vi "AddTestSuite_NoParent_AddedToRoot.vi"() -> (0 "error out":errorcluster)   [LabVIEW 2019, in "ResultTreeTest.lvlib"]
uses:
  ResultTreeTest.lvlib
  2a6c7ef5-d8ea-4de4-ba7d-c6663dbf2225.vi
  Constraint/IsEqual/Create.vi
  Constraint/IsEqual/IsEqual.lvclass
  ResultTree/ResultTree.lvclass
panel:
  in  "Tree":string(tree)
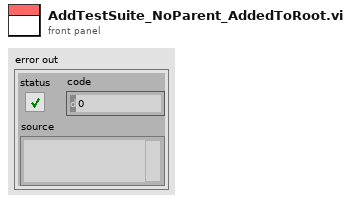
[diagram p1: front panel]
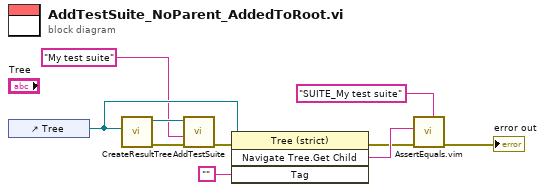
[diagram p0: block diagram]
diagram:
  n1 = control-ref of="Tree"() -> (w9:refnum<vi>)
  n2 = call "CreateResultTree.vi"("Tree Refnum"=w9) -> ("error out"=w8:errorcluster, "ResultTree out"=w6:refnum<class "ResultTree.lvclass">)  [unwired: 9 in]
  n3 = call "AddTestSuite.vi"("error in (no error)"=w8, "Name"="My test suite", "ResultTree in"=w6) -> ("error out"=w7:errorcluster)  [unwired: 6 in, 2 out]
  n4 = invoke class="Tree (strict)" method="Navigate Tree.Get Child"(reference=w9, error in=w7, "Tag"="") -> (error out=w3:errorcluster, "Navigate Tree:Get Child"=w4:string)  [unwired: 1 in, 2 out]
  n5 = call "AssertEquals.vim"("Expected"="SUITE_My test suite" ("Name"), "error in (no error)"=w3, "Actual"=w4) -> ("error out"=→"error out":errorcluster)  [unwired: 8 in]
